vi "Vision Processing.vi"(4 "error in (no error)":errorcluster, 7 "Image Size":T2=enum."320x240") -> ()   [LabVIEW 2013]
doc: "This VI runs in parallel to other tasks. It gets images from the camera, processes them for color or shape and use that information to affect robot behavior."
uses:
  <vilib>/Rock Robotics/WPI/Camera/WPI_CameraImageSize.ctl
  <vilib>/Rock Robotics/WPI/Camera/WPI_CameraWhite Balance Values.ctl
  <vilib>/Rock Robotics/WPI/Camera/WPI_CameraExposure Values.ctl
  <vilib>/Rock Robotics/WPI/Camera/WPI_CameraFrameRate.ctl
  <vilib>/vision/Image Controls.llb/IMAQ Image.ctl
  Robot Global Data.vi
  <vilib>/vision/NI_Vision_Development_Module.lvlib
panel:
  out "Hot Goal/ Side":u32
  out "Image":T1(plugin-control)
  out "error out":errorcluster
  out "True = Left\nFalse = Right":bool
  out "Original":T1(plugin-control)
  out "Hot Goal?":bool
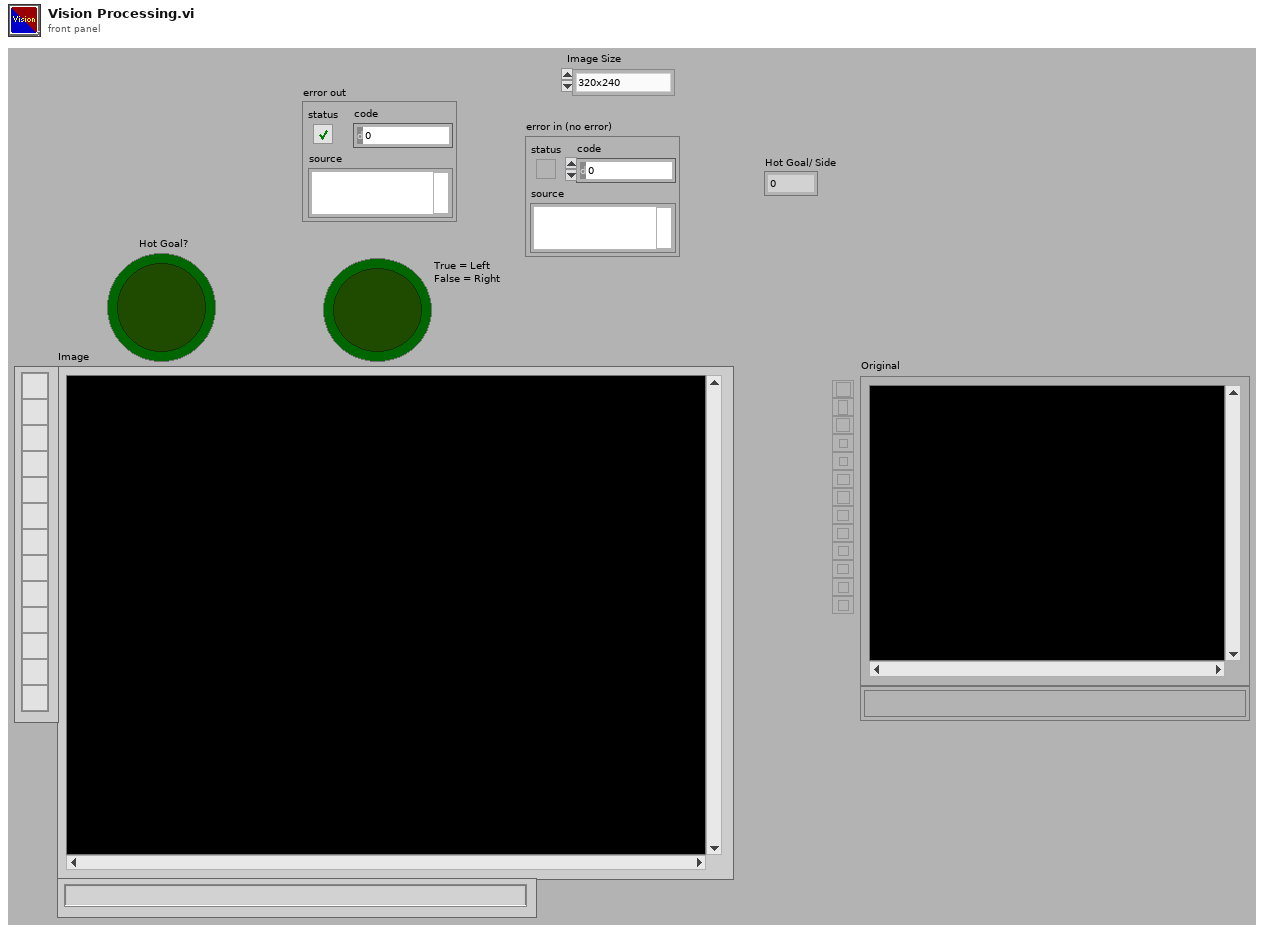
[diagram p1: front panel]
types:
  T1 = typedef "IMAQ Image.ctl" = refnum<image>
  T2 = typedef "WPI_CameraImageSize.ctl" = enum16{"640x480", "320x240", "160x120"}
  T3 = typedef "WPI_CameraFrameRate.ctl" = u32
  T4 = typedef "WPI_CameraExposure Values.ctl" = enum16{"Auto", "Flicker-free 50 Hz", "Flicker-free 60 Hz", "Hold current"}
  T5 = typedef "WPI_CameraWhite Balance Values.ctl" = enum16{"Auto", "Fixed indoor", "Fixed outdoor 1", "Fixed outdoor 2", "Fixed fluorescent 1", "Fixed fluorescent 2", "Hold current"}
  T6 = typedef "Image Type" = u32
  T7 = typedef "WPI_CameraDevRef.ctl" = cluster{"Camera Address":string, "CameraStatus":errorcluster, "Acquire Image Notifier":refnum<notifier>}
  T8 = enum32{"AutoM", "Close", "Dilate", "Erode", "Gradient", "Gradient in", "Gradient out", "HitMiss", "Open", "PClose", "POpen", "Thick", "Thin"}
  T9 = typedef "Particle Parameters" = i32
  T10 = cluster{"Particle Measurements (Pixels)[0]":dbl, "Particle Measurements (Pixels)[1]":dbl}
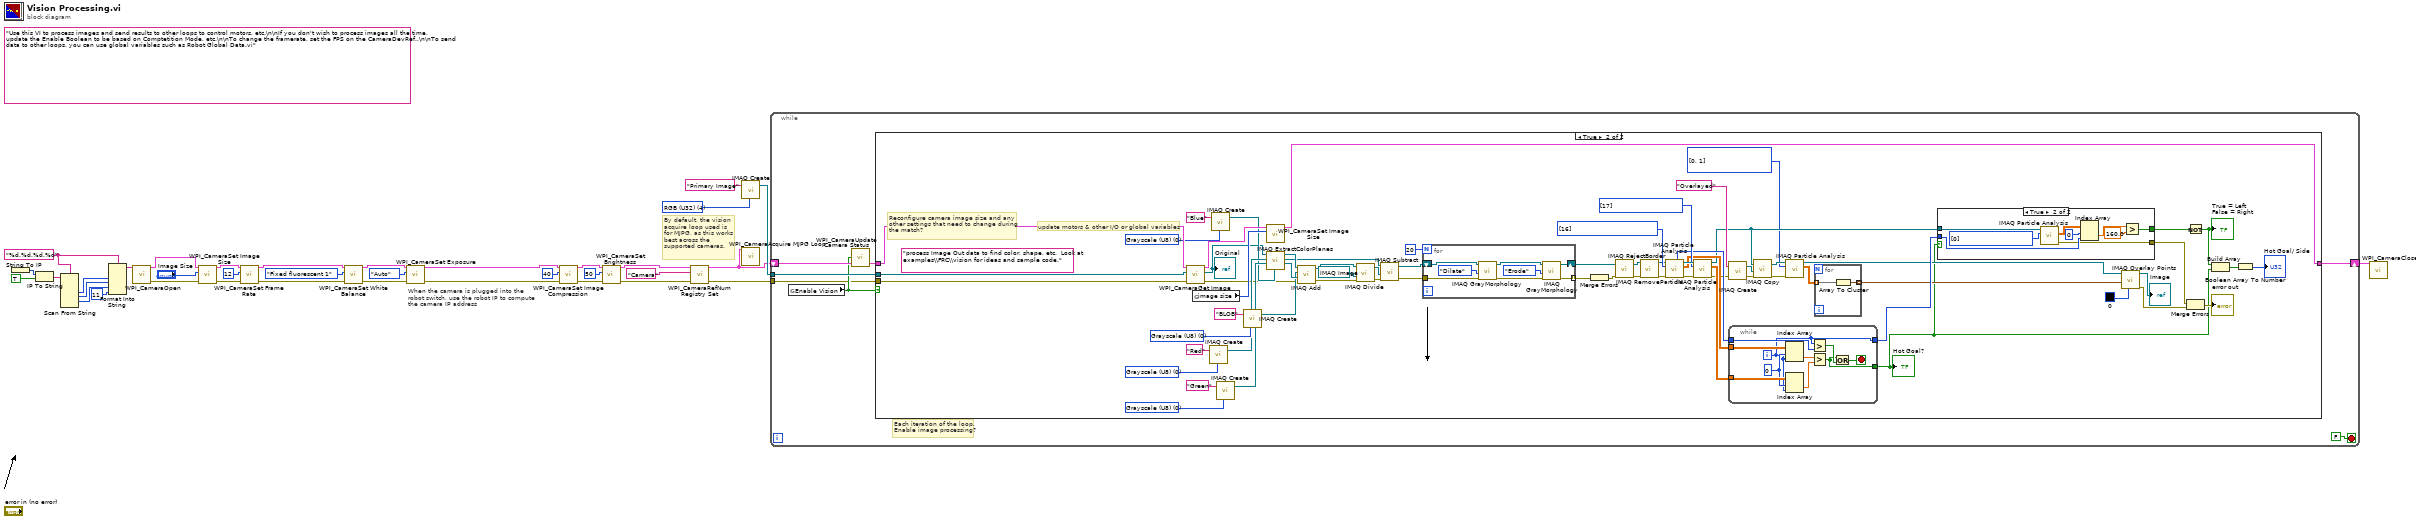
[diagram p0: block diagram]
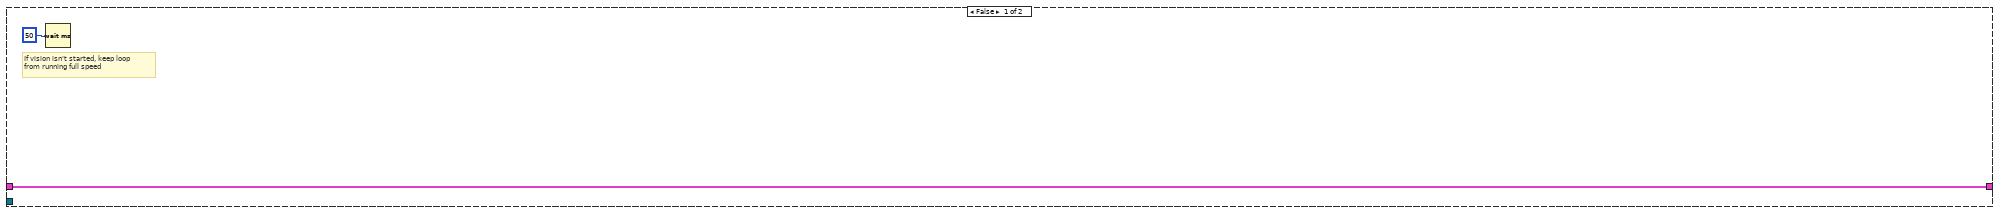
[diagram p2: hidden frame]
diagram:
  w6 = "%d.%d.%d.%d" ("format string")
  (unwired) "Use this VI to process images and send results to other loops to control motors, etc.\n\nIf you don't wish to process images all the time, update the Enable Boolean to be based on Comptetition Mode, etc.\n\nTo change the framerate, set the FPS on the CameraDevRef..\n\nTo send data to other loops, you can use global variables such as Robot Global Data.vi"
  w36 = T6 4 items=["Grayscale (U8)", "Grayscale (I16)", "Grayscale (SGL)", "Complex (CSG)", "RGB (U32)", "HSL (U32)", "RGB (U64)"] ("Image Type")
  # "When the camera is plugged into the\nrobot switch, use the robot IP to compute\nthe camera IP address"
  # "By default, the vision\nacquire loop used is\nfor MJPG, as this works\nbest across the\nsupported cameras."
  n1 = String To IP() -> (0:w13:u32)  [unwired: 1 in]
  n2 = IP To String(1:TRUE ("dot notation? (F)"), 2:w13) -> (0:w11:string)
  n3 = Scan From String(format string=w6, input string=w11) -> (output 1=w10:i32, output 2=w9:i32, output 3=w8:i32)  [unwired: 7 in, 3 out]
  n4 = Format Into String(format string=w6, w10, w9, w8, 11 ("Compression")) -> (resulting string=w5:string)  [unwired: 2 in, 1 out]
  n5 = call <vilib>:"WPI_CameraOpen.vi"("Camera Address"=w5) -> ("error out"=w24:errorcluster, "CameraDevRef"=w25:T7)  [unwired: 1 in, 8 out]
  n6 = call <vilib>:"WPI_CameraSet Image Size.vi"("error in (no error)"=w24, "Image Size"="Image Size", "CameraDevRef"=w25) -> ("error out"=w23:errorcluster, "CameraDevRef Out"=w26:T7)  [unwired: 7 out]
  n7 = call <vilib>:"WPI_CameraSet Frame Rate.vi"("error in (no error)"=w23, "Frame Rate (fps)"=T3 12, "CameraDevRef"=w26) -> ("error out"=w22:errorcluster, "CameraDevRef Out"=w28:T7)  [unwired: 7 out]
  n8 = call <vilib>:"WPI_CameraSet White Balance.vi"("error in (no error)"=w22, "White Balance"=WPI_CameraWhite_Balance_Values."Fixed fluorescent 1", "CameraDevRef"=w28) -> ("error out"=w21:errorcluster, "CameraDevRef Out"=w27:T7)  [unwired: 7 out]
  n9 = call <vilib>:"WPI_CameraSet Exposure.vi"("error in (no error)"=w21, "Exposure"=WPI_CameraExposure_Values."Auto", "CameraDevRef"=w27) -> ("error out"=w20:errorcluster, "CameraDevRef Out"=w30:T7)  [unwired: 7 out]
  n10 = call <vilib>:"WPI_CameraSet Image Compression.vi"("error in (no error)"=w20, "Compression"=40, "CameraDevRef"=w30) -> ("error out"=w19:errorcluster, "CameraDevRef Out"=w29:T7)  [unwired: 7 out]
  n11 = call <vilib>:"WPI_CameraSet Brightness.vi"("error in (no error)"=w19, "Brightness"=50, "CameraDevRef"=w29) -> ("error out"=w17:errorcluster, "CameraDevRef Out"=w18:T7)  [unwired: 7 out]
  n12 = call <vilib>:"WPI_CameraRefNum Registry Set.vi"("error in (no error)"=w17, "refnum name"="Camera", "CameraDevRef"=w18) -> ("error out"=w1:errorcluster, "CameraDevRef"=w4:T7)  [unwired: 7 out]
  n13 = call "IMAQ Create"("Image Name"="Primary Image", "Image Type"=w36) -> ("New Image"=w34:T1)  [unwired: 2 in, 2 out]
  n14 = call <vilib>:"WPI_CameraAcquire MJPG Loop.vi"("CameraDevRef"=w4) -> ()  [unwired: 11 in]
  n15 = while {
    shift-right: [w42] -> w2
    shift-left: w4 -> [w40]
    tunnel: w34 -> [w41]
    tunnel: w1 -> [w37]
    stop <- FALSE stop-if-true
    # "Each iteration of the loop,\nEnable image processing?"
    n16 = global read "Robot Global Data.vi" "Enable Vision"() -> (w38:bool)
    n17 = call <vilib>:"WPI_CameraUpdate Camera Status.vi"("CameraDevRef In"=w40, "Enable Vision"=w38) -> ("CameraDevRef Out"=w39:T7)  [unwired: 3 in]
    n18 = case shown="True" w38 {
      tunnel: w41 -> [_ w111]
      tunnel: [w45 w112] -> w42
      tunnel: w39 -> [w45 w109]
      tunnel: w37 -> [_ w51]
      frame False {
        # "If vision isn't started, keep loop\nfrom running full speed"
        n19 = Wait (ms)(milliseconds to wait=u32 50) -> ()  [unwired: 1 out]
      }
      frame True {
        w57 = T9[] [0, 1] items=["Center of Mass X", "Center of Mass Y", "First Pixel X", "First Pixel Y", "Bounding Rect Left", "Bounding Rect Top", "Bounding Rect Right", "Bounding Rect Bottom", "Max Feret Diameter Start X", "Max Feret Diameter Start Y", "Max Feret Diameter End X", "Max Feret Diameter End Y", "Max Horiz. Segment Length Left", "Max Horiz. Segment Length Right", "Max Horiz. Segment Length Row", "-", "Bounding Rect Width", "Bounding Rect Height", "Bounding Rect Diagonal", "Perimeter", "Convex Hull Perimeter", "Holes' Perimeter", "Max Feret Diameter", "Equivalent Ellipse Major Axis", "Equivalent Ellipse Minor Axis", "Equivalent Ellipse Minor Axis (Feret)", "Equivalent Rect Long Side", "Equivalent Rect Short Side", "Equivalent Rect Diagonal", "Equivalent Rect Short Side (Feret)", "Average Horiz. Segment Length", "Average Vert. Segment Length", "Hydraulic Radius", "Waddel Disk Diameter", "-", "Area", "Holes' Area", "Particle & Holes' Area", "Convex Hull Area", "Image Area", "-", "Number of Holes", "Number of Horiz. Segments", "Number of Vert. Segments", "-", "Orientation", "Max Feret Diameter Orientation", "-", "% Area/Image Area", "% Area/(Particle & Holes' Area)", "Ratio of Equivalent Ellipse Axes", "Ratio of Equivalent Rect Sides", "-", "Elongation Factor", "Compactness Factor", "Heywood Circularity Factor", "Type Factor", "-", "Sum X", "Sum Y", "Sum XX", "Sum XY", "Sum YY", "Sum XXX", "Sum XXY", "Sum XYY", "Sum YYY", "-", "Moment of Inertia XX", "Moment of Inertia XY", "Moment of Inertia YY", "Moment of Inertia XXX", "Moment of Inertia XXY", "Moment of Inertia XYY", "Moment of Inertia YYY", "Norm. Moment of Inertia XX", "Norm. Moment of Inertia XY", "Norm. Moment of Inertia YY", "Norm. Moment of Inertia XXX", "Norm. Moment of Inertia XXY", "Norm. Moment of Inertia XYY", "Norm. Moment of Inertia YYY", "Hu Moment 1", "Hu Moment 2", "Hu Moment 3", "Hu Moment 4", "Hu Moment 5", "Hu Moment 6", "Hu Moment 7"] ("Pixel Measurements")
        w91 = T6 0 items=["Grayscale (U8)", "Grayscale (I16)", "Grayscale (SGL)", "Complex (CSG)", "RGB (U32)", "HSL (U32)", "RGB (U64)", "Grayscale (U16)"] ("Image Type")
        w94 = T6 0 items=["Grayscale (U8)", "Grayscale (I16)", "Grayscale (SGL)", "Complex (CSG)", "RGB (U32)", "HSL (U32)", "RGB (U64)", "Grayscale (U16)"] ("Image Type")
        w96 = T6 0 items=["Grayscale (U8)", "Grayscale (I16)", "Grayscale (SGL)", "Complex (CSG)", "RGB (U32)", "HSL (U32)", "RGB (U64)", "Grayscale (U16)"] ("Image Type")
        w103 = T9[] [17] items=["Center of Mass X", "Center of Mass Y", "First Pixel X", "First Pixel Y", "Bounding Rect Left", "Bounding Rect Top", "Bounding Rect Right", "Bounding Rect Bottom", "Max Feret Diameter Start X", "Max Feret Diameter Start Y", "Max Feret Diameter End X", "Max Feret Diameter End Y", "Max Horiz. Segment Length Left", "Max Horiz. Segment Length Right", "Max Horiz. Segment Length Row", "-", "Bounding Rect Width", "Bounding Rect Height", "Bounding Rect Diagonal", "Perimeter", "Convex Hull Perimeter", "Holes' Perimeter", "Max Feret Diameter", "Equivalent Ellipse Major Axis", "Equivalent Ellipse Minor Axis", "Equivalent Ellipse Minor Axis (Feret)", "Equivalent Rect Long Side", "Equivalent Rect Short Side", "Equivalent Rect Diagonal", "Equivalent Rect Short Side (Feret)", "Average Horiz. Segment Length", "Average Vert. Segment Length", "Hydraulic Radius", "Waddel Disk Diameter", "-", "Area", "Holes' Area", "Particle & Holes' Area", "Convex Hull Area", "Image Area", "-", "Number of Holes", "Number of Horiz. Segments", "Number of Vert. Segments", "-", "Orientation", "Max Feret Diameter Orientation", "-", "% Area/Image Area", "% Area/(Particle & Holes' Area)", "Ratio of Equivalent Ellipse Axes", "Ratio of Equivalent Rect Sides", "-", "Elongation Factor", "Compactness Factor", "Heywood Circularity Factor", "Type Factor", "-", "Sum X", "Sum Y", "Sum XX", "Sum XY", "Sum YY", "Sum XXX", "Sum XXY", "Sum XYY", "Sum YYY", "-", "Moment of Inertia XX", "Moment of Inertia XY", "Moment of Inertia YY", "Moment of Inertia XXX", "Moment of Inertia XXY", "Moment of Inertia XYY", "Moment of Inertia YYY", "Norm. Moment of Inertia XX", "Norm. Moment of Inertia XY", "Norm. Moment of Inertia YY", "Norm. Moment of Inertia XXX", "Norm. Moment of Inertia XXY", "Norm. Moment of Inertia XYY", "Norm. Moment of Inertia YYY", "Hu Moment 1", "Hu Moment 2", "Hu Moment 3", "Hu Moment 4", "Hu Moment 5", "Hu Moment 6", "Hu Moment 7"] ("Pixel Measurements")
        w105 = T9[] [16] items=["Center of Mass X", "Center of Mass Y", "First Pixel X", "First Pixel Y", "Bounding Rect Left", "Bounding Rect Top", "Bounding Rect Right", "Bounding Rect Bottom", "Max Feret Diameter Start X", "Max Feret Diameter Start Y", "Max Feret Diameter End X", "Max Feret Diameter End Y", "Max Horiz. Segment Length Left", "Max Horiz. Segment Length Right", "Max Horiz. Segment Length Row", "-", "Bounding Rect Width", "Bounding Rect Height", "Bounding Rect Diagonal", "Perimeter", "Convex Hull Perimeter", "Holes' Perimeter", "Max Feret Diameter", "Equivalent Ellipse Major Axis", "Equivalent Ellipse Minor Axis", "Equivalent Ellipse Minor Axis (Feret)", "Equivalent Rect Long Side", "Equivalent Rect Short Side", "Equivalent Rect Diagonal", "Equivalent Rect Short Side (Feret)", "Average Horiz. Segment Length", "Average Vert. Segment Length", "Hydraulic Radius", "Waddel Disk Diameter", "-", "Area", "Holes' Area", "Particle & Holes' Area", "Convex Hull Area", "Image Area", "-", "Number of Holes", "Number of Horiz. Segments", "Number of Vert. Segments", "-", "Orientation", "Max Feret Diameter Orientation", "-", "% Area/Image Area", "% Area/(Particle & Holes' Area)", "Ratio of Equivalent Ellipse Axes", "Ratio of Equivalent Rect Sides", "-", "Elongation Factor", "Compactness Factor", "Heywood Circularity Factor", "Type Factor", "-", "Sum X", "Sum Y", "Sum XX", "Sum XY", "Sum YY", "Sum XXX", "Sum XXY", "Sum XYY", "Sum YYY", "-", "Moment of Inertia XX", "Moment of Inertia XY", "Moment of Inertia YY", "Moment of Inertia XXX", "Moment of Inertia XXY", "Moment of Inertia XYY", "Moment of Inertia YYY", "Norm. Moment of Inertia XX", "Norm. Moment of Inertia XY", "Norm. Moment of Inertia YY", "Norm. Moment of Inertia XXX", "Norm. Moment of Inertia XXY", "Norm. Moment of Inertia XYY", "Norm. Moment of Inertia YYY", "Hu Moment 1", "Hu Moment 2", "Hu Moment 3", "Hu Moment 4", "Hu Moment 5", "Hu Moment 6", "Hu Moment 7"] ("Pixel Measurements")
        w106 = T6 0 items=["Grayscale (U8)", "Grayscale (I16)", "Grayscale (SGL)", "Complex (CSG)", "RGB (U32)", "HSL (U32)", "RGB (U64)", "Grayscale (U16)"] ("Image Type")
        (unwired) "process Image Out data to find color, shape, etc.  Look at examples\\FRC\\vision for ideas and sample code."
        # "update motors & other I/O or global variables"
        # "Reconfigure camera image size and any\nother settings that need to change during\nthe match?"
        n20 = call <vilib>:"WPI_CameraGet Image.vi"("error in (no error)"=w51, "Image"=w111, "CameraDevRef"=w109) -> ("error out"=w50:errorcluster, "Image Out"=w52:T1, "CameraDevRef Out"=w108:T7)  [unwired: 6 out]
        "Original" <- w52
        n21 = global read "Robot Global Data.vi" "image size"() -> (w110:T2)
        n22 = call "IMAQ Create"("Image Name"="Red", "Image Type"=w96) -> ("New Image"=w97:T1)  [unwired: 3 in, 1 out]
        n23 = call "IMAQ Create"("Image Name"="Blue", "Image Type"=w91) -> ("New Image"=w90:T1)  [unwired: 3 in, 1 out]
        n24 = call "IMAQ Create"("Image Name"="Green", "Image Type"=w94) -> ("New Image"=w93:T1)  [unwired: 3 in, 1 out]
        n25 = call "IMAQ Create"("Image Name"="BLOB", "Image Type"=w106) -> ("New Image"=w87:T1)  [unwired: 3 in, 1 out]
        n26 = call <vilib>:"WPI_CameraSet Image Size.vi"("Image Size"=w110, "CameraDevRef"=w108) -> ("CameraDevRef Out"=w112:T7)  [unwired: 1 in, 8 out]
        n27 = call "IMAQ ExtractColorPlanes"("Blue or Luma or Val or Inten Plane"=w90, "Green or Sat Plane"=w93, "Red or Hue Plane"=w97, "Image Src"=w52) -> ("Blue or Luma or Val or Inten Plane out"=w88:T1, "Green or Sat Plane out"=w86:T1, "Red or Hue Plane out"=w89:T1)  [unwired: 4 in, 1 out]
        n28 = call "IMAQ Add"("Image Src A"=w89, "Image Dst"=w87, "Image Src B"=w88, "error in (no error)"=w50) -> ("Image Dst Out"=w71:T1, "error out"=w69:errorcluster)  [unwired: 3 in]
        n29 = call "IMAQ Divide"("Image Src A"=w71, "Image Src B"=T1 refnum, "error in (no error)"=w69) -> ("Image Dst Out"=w67:T1, "error out"=w68:errorcluster)  [unwired: 4 in]
        n30 = call "IMAQ Subtract"("Image Src A"=w86, "Image Src B"=w67, "error in (no error)"=w68) -> ("Image Dst Out"=w84:T1, "error out"=w80:errorcluster)  [unwired: 4 in]
        n31 = for {
          N: 20 -> [_]
          shift-right: [w118] -> w83
          shift-left: w84 -> [w119]
          tunnel: w80 -> [w117]
          tunnel: [w115] -> w79 mode=indexing
          n32 = call "IMAQ GrayMorphology"("error in (no error)"=w117, "Operation"=T8."Dilate", "Image Src"=w119) -> ("error out"=w116:errorcluster, "Image Dst Out"=w120:T1)  [unwired: 7 in]
          n33 = call "IMAQ GrayMorphology"("error in (no error)"=w116, "Operation"=T8."Erode", "Image Src"=w120) -> ("error out"=w115:errorcluster, "Image Dst Out"=w118:T1)  [unwired: 7 in]
        }
        n34 = Merge Errors(w79) -> (w78:errorcluster)
        n35 = call "IMAQ RejectBorder"("error in (no error)"=w78, "Image Src"=w83) -> ("error out"=w81:errorcluster, "Image Dst Out"=w82:T1)  [unwired: 4 in]
        n36 = call "IMAQ RemoveParticle"("error in (no error)"=w81, "Image Src"=w82) -> ("error out"=w72:errorcluster, "Image Dst Out"=w73:T1)  [unwired: 8 in]
        n37 = call "IMAQ Particle Analysis"("error in (no error)"=w72, "Pixel Measurements"=w105, "Image"=w73) -> ("error out"=w77:errorcluster, "Particle Measurements (Pixels)"=w102:dbl[][], "Image Out (duplicate)"=w104:T1, "Number of Particles"=w100:i32)  [unwired: 3 in, 2 out]
        n38 = call "IMAQ Particle Analysis"("error in (no error)"=w77, "Pixel Measurements"=w103, "Image"=w104) -> ("error out"=w61:errorcluster, "Particle Measurements (Pixels)"=w101:dbl[][], "Image Out (duplicate)"=w64:T1)  [unwired: 3 in, 3 out]
        n39 = call "IMAQ Create"("Image Name"="Overlayed", "error in (no error)"=w61) -> ("New Image"=w65:T1, "error out"=w60:errorcluster)  [unwired: 3 in]
        n40 = while {
          tunnel: w102 -> [w140]
          tunnel: w101 -> [w141]
          tunnel: w100 -> [w134]
          tunnel: [w133] -> w49
          tunnel: [w132] -> w99
          i -> [w132]
          stop <- w135 stop-if-true
          w139 = 0 ("disabled index (row)")
          n41 = Index Array(array=w140, index (row)=w139, index (col)=w132) -> (element=w137:dbl)
          n42 = Index Array(array=w141, index (row)=w139, index (col)=w132) -> (element=w138:dbl)
          n43 = Greater?(x=w132, y=w134) -> (0:w136:bool)
          n44 = Greater?(x=w137, y=w138) -> (0:w133:bool)
          n45 = Or(x=w133, y=w136) -> (x .or. y?=w135:bool)
        }
        "Hot Goal?" <- w49
        n46 = call "IMAQ Copy"("error in (no error)"=w60, "Image Dst"=w65, "Image Src"=w64) -> ("error out"=w59:errorcluster, "Image Dst Out"=w58:T1)  [unwired: 3 in]
        n47 = call "IMAQ Particle Analysis"("error in (no error)"=w59, "Pixel Measurements"=w57, "Image"=w58) -> ("Particle Measurements (Pixels)"=w56:dbl[][], "Image Out (duplicate)"=w54:T1)  [unwired: 3 in, 4 out]
        n48 = for {
          tunnel: w56 -> [w114] mode=indexing
          tunnel: [w113] -> w55 mode=indexing
          n49 = Array To Cluster(array=w114) -> (cluster=w113:T10)
        }
        n50 = case shown="True" w49 {
          tunnel: w99 -> [_ w127]
          tunnel: w64 -> [_ w130]
          tunnel: [_ w124] -> w74
          tunnel: [_ w123] -> w76
          frame False {
          }
          frame True {
            w131 = T9[] [0] items=["Center of Mass X", "Center of Mass Y", "First Pixel X", "First Pixel Y", "Bounding Rect Left", "Bounding Rect Top", "Bounding Rect Right", "Bounding Rect Bottom", "Max Feret Diameter Start X", "Max Feret Diameter Start Y", "Max Feret Diameter End X", "Max Feret Diameter End Y", "Max Horiz. Segment Length Left", "Max Horiz. Segment Length Right", "Max Horiz. Segment Length Row", "-", "Bounding Rect Width", "Bounding Rect Height", "Bounding Rect Diagonal", "Perimeter", "Convex Hull Perimeter", "Holes' Perimeter", "Max Feret Diameter", "Equivalent Ellipse Major Axis", "Equivalent Ellipse Minor Axis", "Equivalent Ellipse Minor Axis (Feret)", "Equivalent Rect Long Side", "Equivalent Rect Short Side", "Equivalent Rect Diagonal", "Equivalent Rect Short Side (Feret)", "Average Horiz. Segment Length", "Average Vert. Segment Length", "Hydraulic Radius", "Waddel Disk Diameter", "-", "Area", "Holes' Area", "Particle & Holes' Area", "Convex Hull Area", "Image Area", "-", "Number of Holes", "Number of Horiz. Segments", "Number of Vert. Segments", "-", "Orientation", "Max Feret Diameter Orientation", "-", "% Area/Image Area", "% Area/(Particle & Holes' Area)", "Ratio of Equivalent Ellipse Axes", "Ratio of Equivalent Rect Sides", "-", "Elongation Factor", "Compactness Factor", "Heywood Circularity Factor", "Type Factor", "-", "Sum X", "Sum Y", "Sum XX", "Sum XY", "Sum YY", "Sum XXX", "Sum XXY", "Sum XYY", "Sum YYY", "-", "Moment of Inertia XX", "Moment of Inertia XY", "Moment of Inertia YY", "Moment of Inertia XXX", "Moment of Inertia XXY", "Moment of Inertia XYY", "Moment of Inertia YYY", "Norm. Moment of Inertia XX", "Norm. Moment of Inertia XY", "Norm. Moment of Inertia YY", "Norm. Moment of Inertia XXX", "Norm. Moment of Inertia XXY", "Norm. Moment of Inertia XYY", "Norm. Moment of Inertia YYY", "Hu Moment 1", "Hu Moment 2", "Hu Moment 3", "Hu Moment 4", "Hu Moment 5", "Hu Moment 6", "Hu Moment 7"] ("Pixel Measurements")
            n51 = call "IMAQ Particle Analysis"("Pixel Measurements"=w131, "Image"=w130) -> ("error out"=w123:errorcluster, "Particle Measurements (Pixels)"=w129:dbl[][])  [unwired: 4 in, 4 out]
            n52 = Index Array(array=w129, index (row)=0, index (col)=w127) -> (element=w126:dbl)
            n53 = Greater?(x=w126, y=160.0) -> (0:w124:bool)
          }
        }
        n54 = call "IMAQ Overlay Points"("Color"=u32 0, "Array of Points"=w55, "Image"=w54) -> ("error out"=w62:errorcluster, "Image Out"=→"Image":T1)  [unwired: 7 in]
        n55 = Not(x=w74) -> (.not. x?=w48:bool)
        "True = Left\nFalse = Right" <- w48
        n56 = Merge Errors(w76, w62) -> (→"error out":errorcluster)
        n57 = Build Array(w48, w49) -> (w47:bool[])
        n58 = Boolean Array To Number(Boolean array=w47) -> (number=→"Hot Goal/ Side":u32)
      }
    }
  }
  n59 = call <vilib>:"WPI_CameraClose.vi"("CameraDevRef"=w2) -> ()  [unwired: 1 in, 10 out]
